vi "Close.vi"(8 "error in":errorcluster, 11 "Power Actual Value in":refnum<class "Power Actual Value.lvclass">) -> (0 "error out":errorcluster, 3 "Power Actual Value out":refnum<class "Power Actual Value.lvclass">)   [LabVIEW 2023, in "Power Actual Value.lvclass"]
uses:
  Power Actual Value.lvclass
  Parents/Actual Value/Actual Value.lvclass
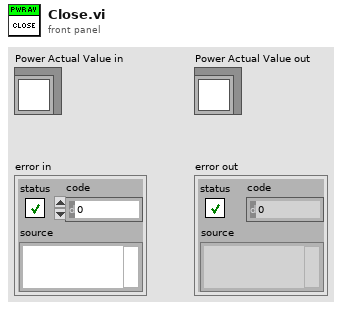
[diagram p1: front panel]
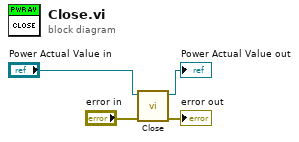
[diagram p0: block diagram]
diagram:
  n1 = call-parent "Close.vi"("error in"="error in", "Actual Value in"="Power Actual Value in") -> ("error out"=→"error out":errorcluster, "Actual Value out"=→"Power Actual Value out":refnum<class "Power Actual Value.lvclass">)  [unwired: 8 in]
